vi "Fitter.vi"(4 "Dly Corr":dbl[](array[numeric]), 6 "Mag Corr":dbl[](array[numeric]), 7 "Window Valid":bool, 8 "error in (no error)":errorcluster, 10 "Test InfoSS":T1={"Fc"=60.0, "Interharmonic"=30.0, "Gen rate"=100000.0, "GenSampls"=1000000, "SmplIntvl s"=5.0, "sampl rate"=48000.0, "sample mode"=10178, "NI Cycles"=3.0, "Delay"=5.0, "Fit Harmonics"=1, "F0"=60.0, "Fs"=60.0} {"sample mode" items=["Finite Samples"=10178, "Continuous Samples"=10123, "Hardware Timed Single Point"=12522]}, 11 "WindowData":T2={"TAI"=3517481187.0499999959, "Data"=array6x2400[14400 elements]} {"TAI" format="%.9f"}) -> (0 "error out":errorcluster, 3 "Phasors":dbl[][](array[numeric]))   [LabVIEW 2014]
uses:
  TypeDefs/SampleData.ctl
  TypeDefs/Test InfoSS.ctl
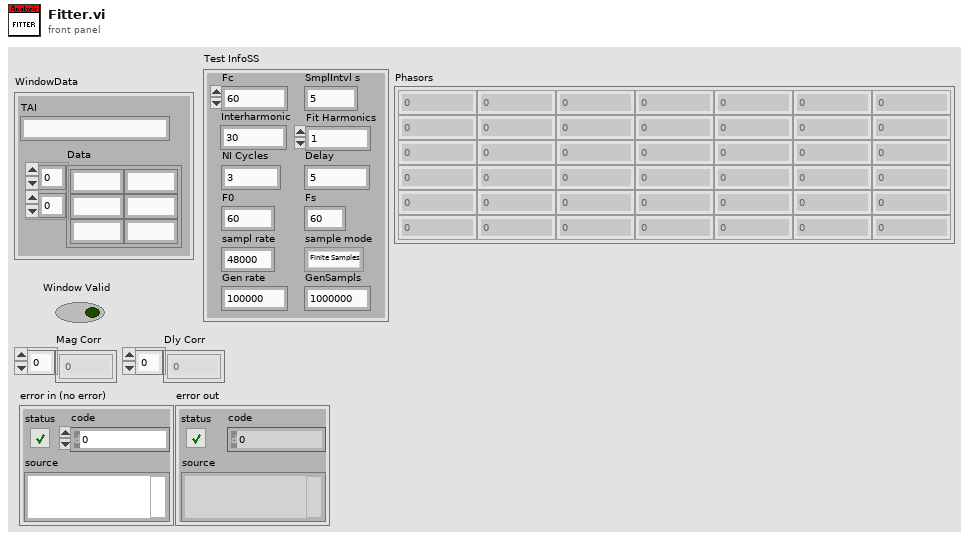
[diagram p1: front panel]
types:
  T1 = typedef "Test InfoSS.ctl" = cluster{"Fc":dbl, "Interharmonic":dbl, "Gen rate":dbl, "GenSampls":i32, "SmplIntvl s":dbl, "sampl rate":dbl, "sample mode":i32, "NI Cycles":dbl, "Delay":dbl, "Fit Harmonics":i32, "F0":dbl, "Fs":dbl}
  T2 = typedef "SampleData.ctl" = cluster{"TAI":ext, "Data":dbl[][]}
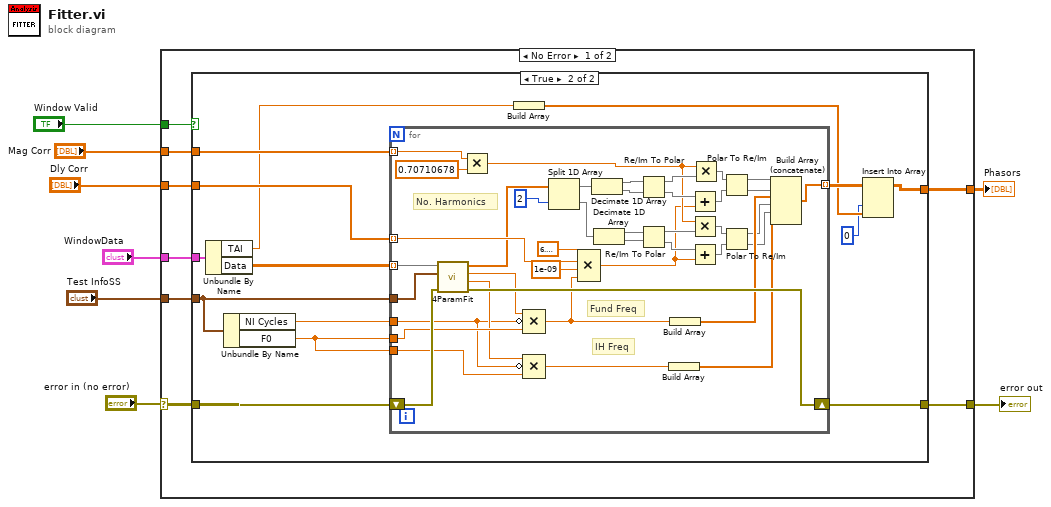
[diagram p0: block diagram]
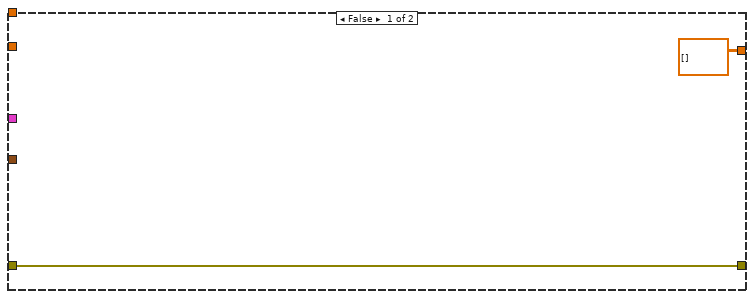
[diagram p2: hidden frame]
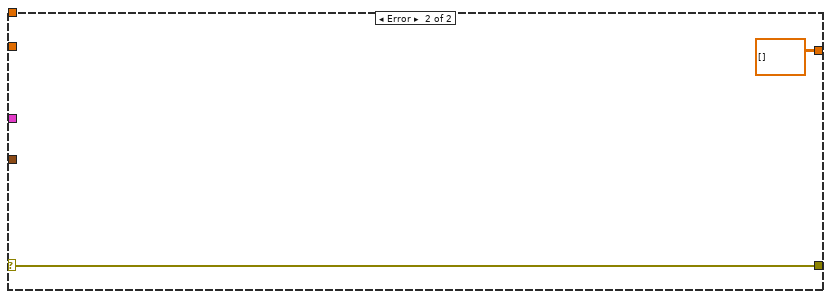
[diagram p3: hidden frame]
diagram:
  n1 = case shown="No Error" "error in (no error)" {
    selector: "error in (no error)" -> [w15 w75]
    tunnel: [w14 w75] -> w7
    tunnel: "WindowData" -> [w16 _]
    tunnel: "Test InfoSS" -> [w13 _]
    tunnel: "Window Valid" -> [w12 _]
    tunnel: "Mag Corr" -> [w11 _]
    tunnel: "Dly Corr" -> [w10 _]
    tunnel: [w9 dbl[][] []] -> w1
    frame No Error {
      n2 = case shown="True" w12 {
        tunnel: w16 -> [_ w32]
        tunnel: w15 -> [w18 w30]
        tunnel: [w18 w29] -> w14
        tunnel: w13 -> [_ w27]
        tunnel: w11 -> [_ w28]
        tunnel: w10 -> [_ w25]
        tunnel: [dbl[][] [] w23] -> w9
        frame False {
        }
        frame True {
          n3 = Unbundle By Name(w32) -> ("TAI"=w22:ext, "Data"=w31:dbl[][])
          n4 = Unbundle By Name(w27) -> ("NI Cycles"=w26:dbl, "F0"=w19:dbl)
          n5 = for {
            tunnel: w31 -> [w73] mode=indexing
            shift-right: [w68] -> w29
            shift-left: w30 -> [w69]
            tunnel: w27 -> [w72]
            tunnel: w28 -> [w70] mode=indexing
            tunnel: w26 -> [w48]
            tunnel: w19 -> [w66]
            tunnel: w25 -> [w62] mode=indexing
            tunnel: [w53] -> w24 mode=indexing
            tunnel: w19 -> [w47]
            # "IH Freq"
            # "Fund Freq"
            # "No. Harmonics"
            n6 = call "4ParamFit.vi"("error in (no error)"=w69, "Test InfoSS"=w72, "Voltage \nSamples"=w73) -> ("error out"=w68:errorcluster, "Interharm Cyc out"=w49:dbl, "Fund Cyc out"=w67:dbl, "Rect Components"=w52:dbl[])  [unwired: 4 in, 1 out]
            n7 = Multiply(x=w70, y=0.70710678) -> (x*y=w41:dbl)
            n8 = Compound Arithmetic op=MULTIPLY(w67, invert w48, w66) -> (w59:dbl)
            n9 = Compound Arithmetic op=MULTIPLY(w49, invert w48, w47) -> (w34:dbl)
            n10 = Split 1D Array(array=w52, index=2 ("length")) -> (first subarray=w46:dbl[], second subarray=w45:dbl[])
            n11 = Compound Arithmetic op=MULTIPLY(6.283185307179586, w62, 1e-09 ("value"), w59) -> (w39:dbl)
            n12 = Decimate 1D Array(w46) -> (w65:dbl[], w64:dbl[])
            n13 = Decimate 1D Array(w45) -> (w44:dbl[], w43:dbl[])
            n14 = Re/Im To Polar(2:w64, 3:w65) -> (0:w58:dbl[], 1:w63:dbl[])
            n15 = Re/Im To Polar(2:w43, 3:w44) -> (0:w40:dbl[], 1:w42:dbl[])
            n16 = Build Array(w34) -> (w33:dbl[])
            n17 = Build Array(w59) -> (w51:dbl[])
            n18 = Add(x=w58, y=w39) -> (x+y=w56:dbl[])
            n19 = Multiply(x=w41, y=w42) -> (x*y=w37:dbl[])
            n20 = Add(x=w40, y=w39) -> (x+y=w38:dbl[])
            n21 = Multiply(x=w41, y=w63) -> (x*y=w57:dbl[])
            n22 = Polar To Re/Im(2:w56, 3:w57) -> (0:w54:dbl[], 1:w55:dbl[])
            n23 = Polar To Re/Im(2:w38, 3:w37) -> (0:w35:dbl[], 1:w36:dbl[])
            n24 = Build Array (concatenate)(w55, w54, w51, w36, w35, w33) -> (w53:dbl[])
          }
          n25 = Build Array(w22) -> (w21:ext[])
          n26 = Insert Into Array(array=w24, index (col)=0 ("disabled index (col)"), new element=w21) -> (w23:dbl[][])  [unwired: 1 in]
        }
      }
    }
    frame Error {
    }
  }
  "error out" <- w7
  "Phasors" <- w1
